vi "GetLinePoints.vi"(10 "Percentage Fill":dbl, 11 "Image":T1) -> (0 "error out":errorcluster, 2 "End Point":cluster{"X":i32, "Y":i32}, 3 "Start Point":cluster{"X":i32, "Y":i32})   [LabVIEW 2024]
uses:
  <vilib>/vision/Image Controls.llb/IMAQ Image.ctl
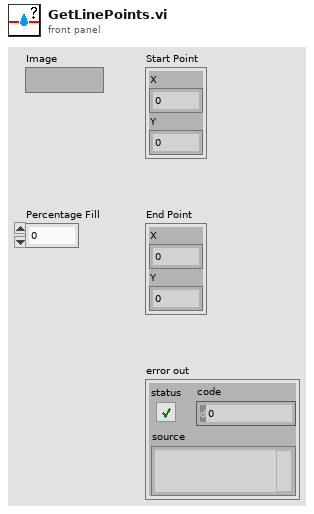
[diagram p1: front panel]
types:
  T1 = typedef "IMAQ Image.ctl" = refnum<image>
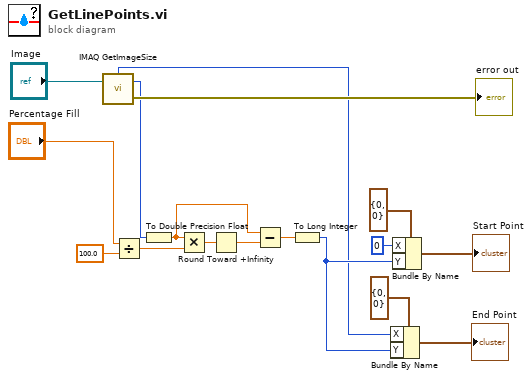
[diagram p0: block diagram]
diagram:
  n1 = call "IMAQ GetImageSize"("Image"="Image") -> ("Y Resolution"=w2:i32, "X Resolution"=w1:i32, "error out"=→"error out":errorcluster)  [unwired: 3 in]
  n2 = Divide(x="Percentage Fill", y=100.0) -> (x/y=w8:dbl)
  n3 = To Double Precision Float(number=w2) -> (double precision float=w7:dbl)
  n4 = Multiply(x=w7, y=w8) -> (x*y=w10:dbl)
  n5 = Round Toward +Infinity(x=w10) -> (ceil(x): smallest int >= x=w9:dbl)
  n6 = Subtract(x=w7, y=w9) -> (x-y=w6:dbl)
  n7 = To Long Integer(number=w6) -> (32bit integer=w3:i32)
  n8 = Bundle By Name(cluster=cluster{"X":i32, "Y":i32} {"X"=0, "Y"=0} ("Start Point"), "X"=w1, "Y"=w3) -> (→"End Point":cluster{"X":i32, "Y":i32})
  n9 = Bundle By Name(cluster=cluster{"X":i32, "Y":i32} {"X"=0, "Y"=0} ("Start Point"), "X"=0, "Y"=w3) -> (→"Start Point":cluster{"X":i32, "Y":i32})
